vi "ReadPhotos.vi"(11 "Path To Instrument Folder":path) -> (1 "zoom":dbl, 3 "photos":picture[](array[picture]))   [LabVIEW 2022 SP3]
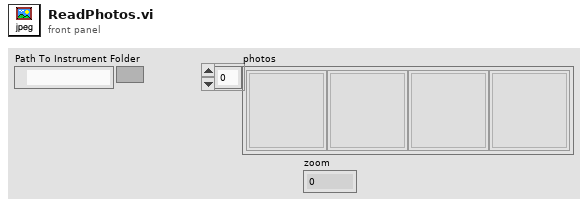
[diagram p1: front panel]
types:
  T1 = typedef "LVBoundsTypeDef.ctl" = cluster{"Width":u32, "Height":u32}
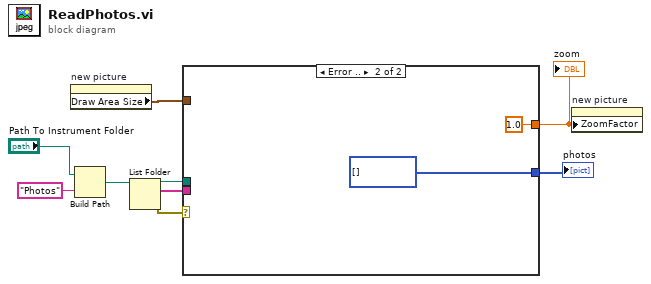
[diagram p0: block diagram]
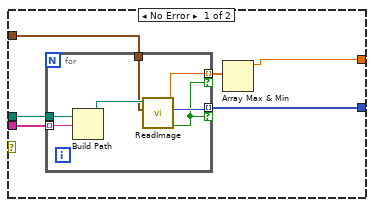
[diagram p2: hidden frame]
diagram:
  n1 = property on="new picture" class="Pict"() -> ("Draw Area Size"=w2:T1)  [unwired: 2 in, 2 out]
  n2 = Build Path(base path="Path To Instrument Folder", name or relative path="Photos") -> (appended path=w7:path)
  n3 = List Folder(path=w7) -> (path out=w5:path, filenames=w4:string[], error out=w3:errorcluster)  [unwired: 3 in, 1 out]
  n4 = case shown="Error .." w3 {
    tunnel: [w15 picture[] []] -> w6
    tunnel: w5 -> [w14 _]
    tunnel: w4 -> [w13 _]
    tunnel: w2 -> [w12 _]
    tunnel: [w10 1.0] -> w1
    frame No Error {
      n5 = for {
        tunnel: [w19] -> w15 mode=indexing if=w16
        tunnel: w14 -> [w22]
        tunnel: w13 -> [w21] mode=indexing
        tunnel: w12 -> [w18]
        tunnel: [w17] -> w11 mode=indexing if=w16
        n6 = Build Path(base path=w22, name or relative path=w21) -> (appended path=w20:path)
        n7 = call "ReadImage.vi"("Draw Area Size"=w18, "Image path"=w20) -> ("success?"=w16:bool, "Image"=w19:picture, "zoom"=w17:dbl)  [unwired: 7 in]
      }
      n8 = Array Max & Min(array=w11) -> (max value=w10:dbl)  [unwired: 3 out]
    }
    frame Error {
    }
  }
  "photos" <- w6
  "zoom" <- w1
  n9 = property on="new picture" class="Pict"("ZoomFactor"=w1) -> ()  [unwired: 2 in, 2 out]
